vi "ErrorHandling.Gui.vi"(5 "~Critical? (T)":bool=TRUE, 6 "~Shutdown visible (T)":bool=TRUE, 7 "~Source":T1, 8 "error in (no error)":errorcluster, 9 "~Action (Calling VI)":string, 10 "Log to disk? (T)":bool=TRUE, 11 "~Show? (T)":bool=TRUE) -> (0 "error out":errorcluster, 2 "~shutdown?":bool)   [LabVIEW 2019, in "Tools.lvlib"]
uses:
  Tools.lvlib
  controls/buttons/Shutdown.ctl
  controls/buttons/OK.ctl
  ErrorHandling.ErrSource.ctl
  ErrorHandling.Gui.Action.ctl
panel:
  out "_loop":i32(ring)=4
  in  "open?":bool
  out "~ErrorMessage":string
  in  "OKButton":T2
  in  "ShutdownButton":T3
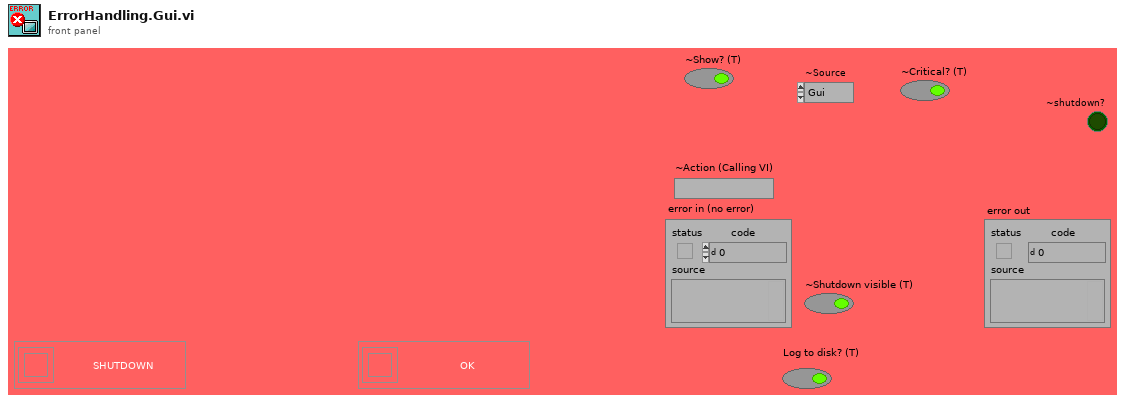
[diagram p1: front panel]
types:
  T1 = typedef "Tools.lvlib/ErrorHandling.ErrSource.ctl" = enum16{"Gui", "Init"}
  T2 = typedef "Tools.lvlib/OK.ctl" = bool
  T3 = typedef "Tools.lvlib/Shutdown.ctl" = bool
  T4 = typedef "Tools.lvlib/ErrorHandling.Gui.Action.ctl" = enum32{"idle", "constructor", "destructor", "--- ErrorGUI ---"}
  T5 = enum32{"Invalid", "Standard", "Closed", "Hidden", "Minimized", "Maximized"}
  T6 = enum32{"invalid app kind", "Development System", "Run Time System", "Student Edition", "Embedded LabVIEW", "Evaluation", "Custom"}
  T7 = typedef "LVPositionTypeDef.ctl" = cluster{"Left":i32, "Top":i32}
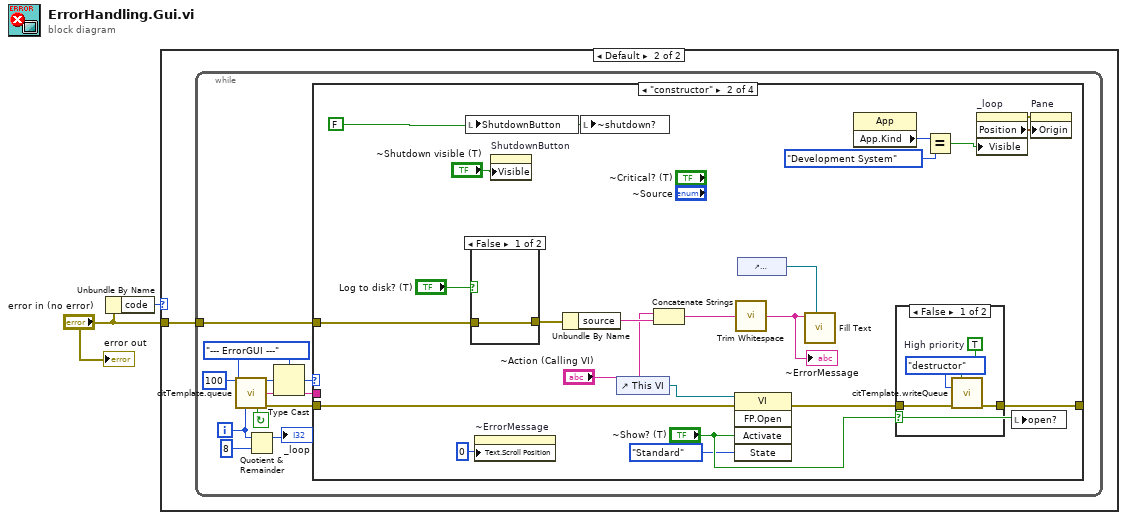
[diagram p0: block diagram]
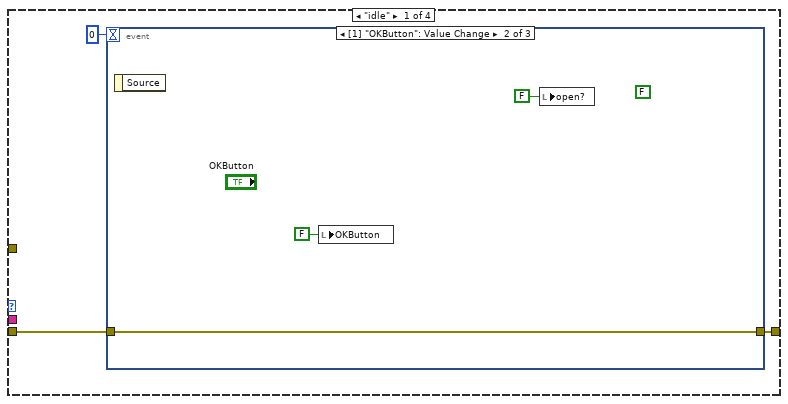
[diagram p3: hidden frame]
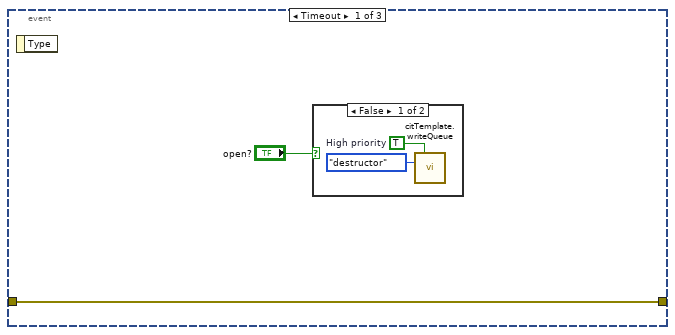
[diagram p4: hidden frame]
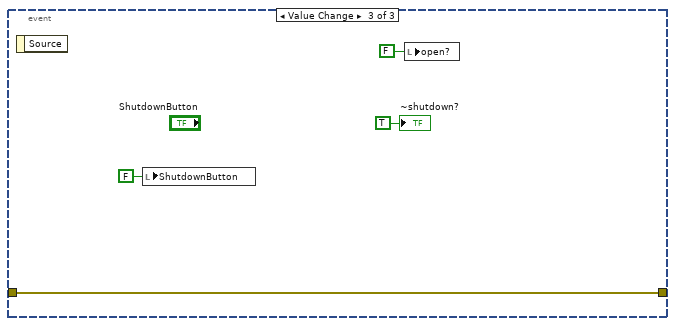
[diagram p6: hidden frame]
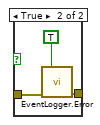
[diagram p7: hidden frame]
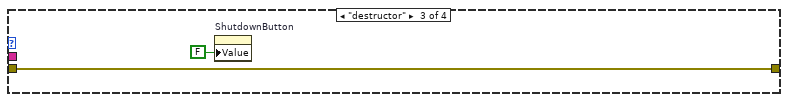
[diagram p9: hidden frame]
diagram:
  n1 = Unbundle By Name("error in (no error)") -> ("code"=w2:i32)
  n2 = case shown="Default" w2 {
    tunnel: "error in (no error)" -> [_ w3]
    frame 0 {
    }
    frame Default {
      n3 = while {
        tunnel: w3 -> [w4]
        i -> [w6]
        stop <- w14 continue-if-true
        w8 = ErrorHandling.Gui.Action."--- ErrorGUI ---" ("Action")
        n4 = call "citTemplate.queue.vi"("ms timeout (250 ms)"=100, "event enum"=w8, "iteration (-1)"=w6) -> ("event out"=w12:u32, "(flatten) data out"=w9:string, "continue"=w14:bool, "error out"=w10:errorcluster)  [unwired: 2 in, 7 out]
        n5 = Quotient & Remainder(x=w6, y=8) -> (x-y*floor(x/y)=→"_loop":i32)  [unwired: 1 out]
        n6 = Type Cast(type=w8, x=w12) -> (*(type *) &x=w11:T4)
        n7 = case shown="\"constructor\"" w11 {
          tunnel: [w15 w39 w61 w62] -> _
          tunnel: w10 -> [w16 w48 w61 w62]
          tunnel: w9 -> [_ _ _ _]
          tunnel: w4 -> [_ w49 _ _]
          frame "idle" {
            n8 = event shown="[1] \"OKButton\": Value Change" {
              selector: _ -> [_ _ _]
              dyn-events: _ -> [_ _ _]
              timeout: 0 -> [_ _ _]
              tunnel: w16 -> [w19 w23 w28]
              tunnel: [w19 w23 w28] -> w15
              event Timeout {
                n9 = event-data() -> ()  [unwired: 2 out]
                n10 = case shown="False" "open?" {
                  frame False {
                    w20 = TRUE  # High priority
                    n11 = call "citTemplate.writeQueue.vi"("High priority (F)"=w20, "event in (if not connected:all statemachine with data event)"=ErrorHandling.Gui.Action."destructor" ("Action")) -> ()  [unwired: 3 in, 11 out]
                  }
                  frame True {
                  }
                }
              }
              event Value Change {
                (unwired) FALSE ("Value (Signaling)")
                n12 = event-data() -> ()  [unwired: 2 out]
                n13 = local write "OKButton"(T2 FALSE ("OKButton")) -> ()
                n14 = local write "open?"(FALSE ("open?")) -> ()
              }
              event Value Change {
                n15 = event-data() -> ()  [unwired: 2 out]
                n16 = local write "ShutdownButton"(T3 FALSE ("ShutdownButton")) -> ()
                n17 = local write "open?"(FALSE ("open?")) -> ()
                "~shutdown?" <- TRUE ("~shutdown?")
              }
            }
          }
          frame "constructor" {
            w44 = FALSE ("Value (Signaling)")
            n18 = local write "ShutdownButton"(w44) -> ()
            n19 = case shown="False" "Log to disk? (T)" {
              tunnel: w49 -> [w51 w54]
              tunnel: [w51 w53] -> w38
              frame False {
              }
              frame True {
                n20 = call "EventLogger.Error.vi"("Flush To Disk On Error"=TRUE, "error in"=w54) -> ("error out"=w53:errorcluster)  [unwired: 9 in]
              }
            }
            n21 = property on="~ErrorMessage" class="Str"("Text.Scroll Position"=u32 0) -> ()  [unwired: 2 in, 2 out]
            n22 = property on="ShutdownButton" class="Bool (strict)"("Visible"="~Shutdown visible (T)") -> ()  [unwired: 2 in, 2 out]
            n23 = Unbundle By Name(w38) -> ("source"=w33:string)
            n24 = local write "~shutdown?"(w44) -> ()
            n25 = control-ref of="This VI"() -> (w31:refnum<vi>)
            n26 = Concatenate Strings("~Action (Calling VI)", w33) -> (w34:string)
            n27 = invoke class="VI" method="FP.Open"(reference=w31, error in=w48, "Activate"="~Show? (T)", "State"=T5."Standard") -> (error out=w47:errorcluster)  [unwired: 1 in, 4 out]
            n28 = call <vilib>:"Trim Whitespace.vi"("string"=w34) -> ("trimmed string"=w37:string)  [unwired: 1 in]
            "~ErrorMessage" <- w37
            n29 = control-ref of="~ErrorMessage"() -> (w36:refnum<vi>)
            n30 = call "Fill Text.vi"("String ref"=w36, "String in"=w37) -> ()  [unwired: 9 in, 1 out]
            n31 = property class="App"() -> ("App.Kind"=w42:T6)  [unwired: 2 in, 2 out]
            n32 = case shown="False" "~Show? (T)" {
              tunnel: w47 -> [w58 w59]
              tunnel: [w57 w59] -> w39
              frame False {
                w55 = TRUE  # High priority
                n33 = call "citTemplate.writeQueue.vi"("High priority (F)"=w55, "event in (if not connected:all statemachine with data event)"=ErrorHandling.Gui.Action."destructor" ("Action"), "error in (no error)"=w58) -> ("error out"=w57:errorcluster)  [unwired: 2 in, 10 out]
              }
              frame True {
              }
            }
            n34 = Equal?(x=w42, y=T6."Development System") -> (x = y?=w40:bool)
            n35 = property on="_loop" class="Ring (strict)"("Visible"=w40) -> (error out=w46:errorcluster, "Position"=w45:T7)  [unwired: 2 in, 1 out]
            n36 = local write "open?"("~Show? (T)") -> ()
            n37 = property on="Pane" class="Pane"(error in=w46, "Origin"=w45) -> ()  [unwired: 1 in, 2 out]
          }
          frame "destructor" {
            n38 = property on="ShutdownButton" class="Bool (strict)"("Value"=FALSE ("ShutdownButton")) -> ()  [unwired: 2 in, 2 out]
          }
          frame "--- ErrorGUI ---" {
          }
        }
      }
    }
  }
  "error out" <- "error in (no error)"
